vi "maximier.vi"(0 "L_k(t)":ext[][](array[numeric]), 1 "H_lk":ext[][][](array[numeric]), 6 "online_ERP_raw":dbl[][](array[numeric]), 7 "STD":dbl[](array[numeric])) -> (14 "covariance_target":dbl[][](array[numeric]), 15 "covariance_nontarget":dbl[][](array[numeric]), 16 "Average_TERP":dbl[](array[numeric]), 17 "Average_NTERP":dbl[](array[numeric]), 19 "akl":ext[][](array[numeric]))   [LabVIEW 2013]
uses:
  <vilib>/Analysis/baseanly.llb/Real A x B.vi
  <vilib>/Analysis/Matrix/Numeric/Conversions/Array To Matrix - RA.vi
  <vilib>/Analysis/Matrix/Numeric/Conversions/Matrix To Array - RM.vi
  <vilib>/Analysis/Matrix/NI_Matrix.lvlib
  <vilib>/Analysis/NI_AALBase.lvlib
panel:
  in  "Tab Control":enum32{"Input", "mu_k", "covariance_k", "alk"}(tab)
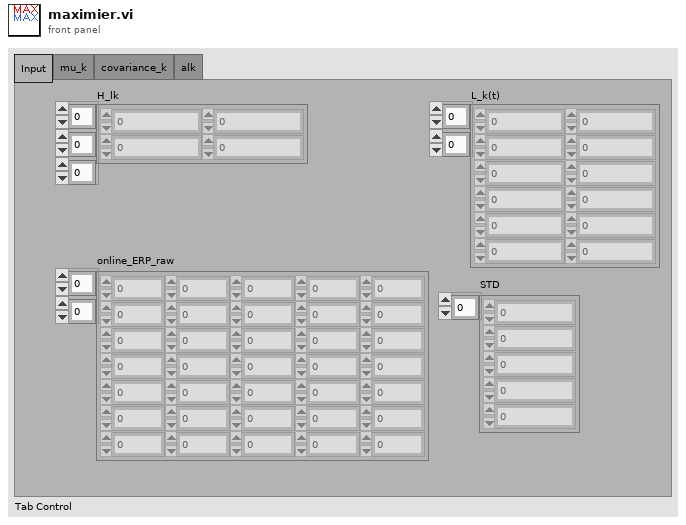
[diagram p1: front panel]
types:
  T1 = typedef "NI_Matrix.lvlib/RealMatrix.ctl" = dbl[][]
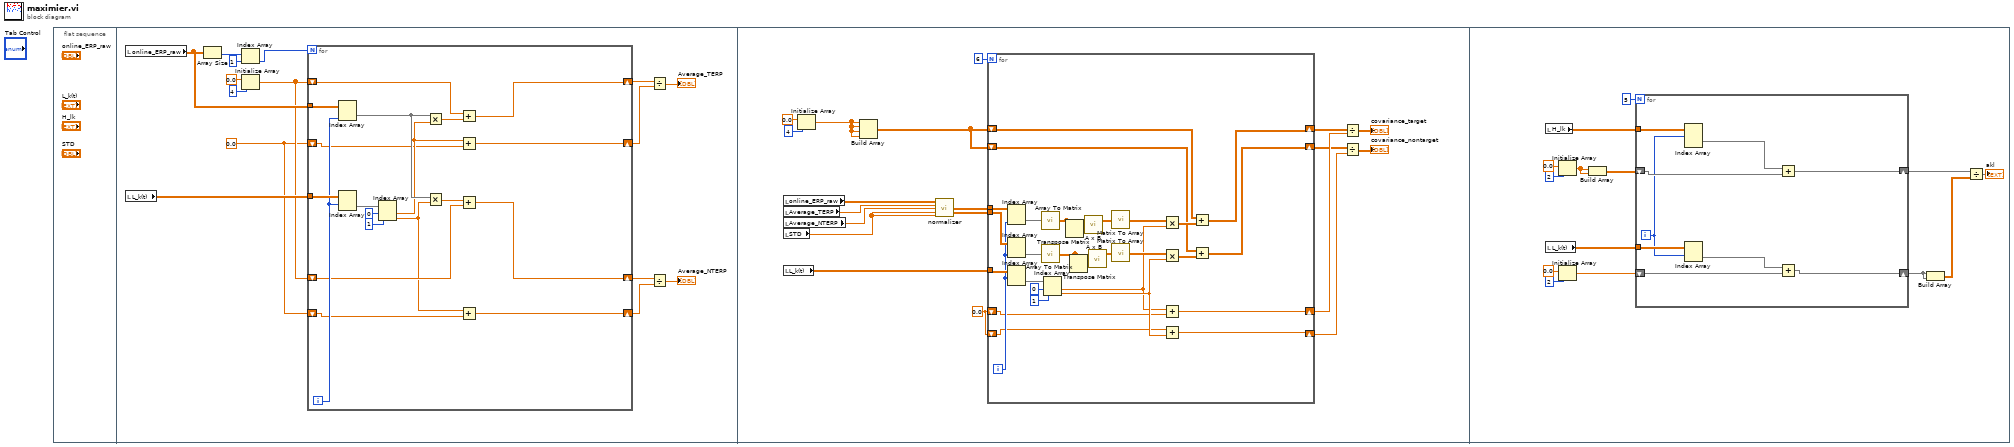
[diagram p0: block diagram]
diagram:
  n1 = flat-sequence {
    frame #0 {
    }
    frame #1 {
      w4 = 0.0
      n2 = local read "online_ERP_raw"() -> (w12:dbl[][])
      n3 = local read "L_k(t)"() -> (w11:ext[][])
      n4 = Array Size(array=w12) -> (size(s)=w15:i32[])
      n5 = Index Array(array=w15, index=1) -> (element=w13:i32)
      n6 = Initialize Array(0.0 ("element"), 4 ("dimension size")) -> (w5:dbl[])
      n7 = for {
        N: w13 -> [_]
        tunnel: w12 -> [w34]
        tunnel: w11 -> [w33]
        shift-right: [w26] -> w8
        shift-left: w5 -> [w25]
        shift-right: [w23] -> w7
        shift-left: w4 -> [w22]
        shift-right: [w20] -> w3
        shift-left: w5 -> [w19]
        shift-right: [w17] -> w2
        shift-left: w4 -> [w16]
        i -> [w31]
        n8 = Index Array(array=w34, index (col)=w31) -> (element=w28:dbl[])  [unwired: 1 in]
        n9 = Index Array(array=w33, index (row)=w31) -> (element=w32:ext[])  [unwired: 1 in]
        n10 = Index Array(array=w32, index #1=0 ("index"), index #2=1 ("index")) -> (element #1=w24:ext, element #2=w18:ext)
        n11 = Multiply(x=w28, y=w24) -> (x*y=w27:ext[])
        n12 = Multiply(x=w28, y=w18) -> (x*y=w21:ext[])
        n13 = Add(x=w25, y=w27) -> (x+y=w26:ext[])
        n14 = Add(x=w24, y=w22) -> (x+y=w23:ext)
        n15 = Add(x=w21, y=w19) -> (x+y=w20:ext[])
        n16 = Add(x=w18, y=w16) -> (x+y=w17:ext)
      }
      n17 = Divide(x=w8, y=w7) -> (x/y=→"Average_TERP":ext[])
      n18 = Divide(x=w3, y=w2) -> (x/y=→"Average_NTERP":ext[])
    }
    frame #2 {
      w45 = 0.0
      n19 = local read "online_ERP_raw"() -> (w53:dbl[][])
      n20 = local read "Average_TERP"() -> (w51:dbl[])
      n21 = local read "Average_NTERP"() -> (w50:dbl[])
      n22 = local read "STD"() -> (w52:dbl[])
      n23 = local read "L_k(t)"() -> (w46:ext[][])
      n24 = Initialize Array(0.0 ("element"), 4 ("dimension size")) -> (w42:dbl[])
      n25 = Build Array(w42, w42, w42, w42) -> (w41:dbl[][])
      n26 = call "normalizer.vi"("online_ERP_raw"=w53, "Average_TERP"=w51, "Average_NTERP"=w50, "STD_TERP"=w52, "STD_NTERP"=w52) -> ("ut_target"=w49:dbl[][], "ut_nontarget"=w48:dbl[][])  [unwired: 9 in]
      n27 = for {
        N: 6 -> [_]
        tunnel: w49 -> [w81]
        tunnel: w48 -> [w80]
        tunnel: w46 -> [w82]
        shift-right: [w63] -> w39
        shift-left: w45 -> [w62]
        shift-right: [w61] -> w37
        shift-left: w45 -> [w60]
        shift-right: [w57] -> w40
        shift-left: w41 -> [w56]
        shift-right: [w55] -> w38
        shift-left: w41 -> [w54]
        i -> [w79]
        n28 = Index Array(array=w81, index (col)=w79) -> (element=w75:dbl[])  [unwired: 1 in]
        n29 = Index Array(array=w80, index (col)=w79) -> (element=w74:dbl[])  [unwired: 1 in]
        n30 = Index Array(array=w82, index (row)=w79) -> (element=w78:ext[])  [unwired: 1 in]
        n31 = call-poly <vilib>:"Array To Matrix.vi"("Real 1D Array"=w75) -> ("Real Matrix (Column Vector)"=w73:T1)
        n32 = call-poly <vilib>:"Array To Matrix.vi"("Real 1D Array"=w74) -> ("Real Matrix (Column Vector)"=w70:T1)
        n33 = Index Array(array=w78, index #1=0 ("index"), index #2=1 ("index")) -> (element #1=w64:ext, element #2=w65:ext)
        n34 = Transpose Matrix(1:w73) -> (0:w72:T1)
        n35 = Transpose Matrix(1:w70) -> (0:w71:T1)
        n36 = call-poly <vilib>:"A x B.vi"("B"=w72, "A"=w73) -> ("A x B"=w69:T1)  [unwired: 1 out]
        n37 = call-poly <vilib>:"A x B.vi"("B"=w71, "A"=w70) -> ("A x B"=w68:T1)  [unwired: 1 out]
        n38 = call-poly <vilib>:"Matrix To Array.vi"("Real Matrix"=w69) -> ("Real 2D Array"=w67:dbl[][])
        n39 = call-poly <vilib>:"Matrix To Array.vi"("Real Matrix"=w68) -> ("Real 2D Array"=w66:dbl[][])
        n40 = Multiply(x=w67, y=w64) -> (x*y=w59:ext[][])
        n41 = Multiply(x=w66, y=w65) -> (x*y=w58:ext[][])
        n42 = Add(x=w64, y=w62) -> (x+y=w63:ext)
        n43 = Add(x=w60, y=w65) -> (x+y=w61:ext)
        n44 = Add(x=w56, y=w59) -> (x+y=w57:ext[][])
        n45 = Add(x=w54, y=w58) -> (x+y=w55:ext[][])
      }
      n46 = Divide(x=w40, y=w39) -> (x/y=→"covariance_target":ext[][])
      n47 = Divide(x=w38, y=w37) -> (x/y=→"covariance_nontarget":ext[][])
    }
    frame #3 {
      n48 = local read "H_lk"() -> (w96:ext[][][])
      n49 = local read "L_k(t)"() -> (w90:ext[][])
      n50 = Initialize Array(0.0 ("element"), 2 ("dimension size")) -> (w92:dbl[])
      n51 = Initialize Array(0.0 ("element"), 2 ("dimension size")) -> (w87:dbl[])
      n52 = Build Array(w92, w92) -> (w91:dbl[][])
      n53 = for {
        N: 5 -> [_]
        tunnel: w96 -> [w105]
        shift-right: [w103] -> w85
        shift-left: w91 -> [w102]
        tunnel: w90 -> [w101]
        shift-right: [w97] -> w86
        shift-left: w87 -> [w98]
        i -> [w100]
        n54 = Index Array(array=w105, index (dim 0)=w100) -> (element=w104:ext[][])  [unwired: 2 in]
        n55 = Index Array(array=w101, index (row)=w100) -> (element=w99:ext[])  [unwired: 1 in]
        n56 = Add(x=w104, y=w102) -> (x+y=w103:ext[][])
        n57 = Add(x=w99, y=w98) -> (x+y=w97:ext[])
      }
      n58 = Build Array(w86, w86) -> (w84:ext[][])
      n59 = Divide(x=w85, y=w84) -> (x/y=→"akl":ext[][])
    }
  }
